vi "horizon_line.vi"(4 "center":cluster{"x":i32, "y":i32}={"x"=51, "y"=51}, 5 "color":u32(colorbox)=16711680, 6 "size":i32=40, 10 "pict in":picture) -> (3 "new out":picture)   [LabVIEW 2011]
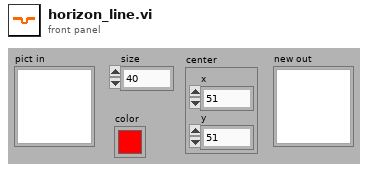
[diagram p1: front panel]
types:
  T1 = cluster{"Width":u16, "Style":enum32{"Solid", "Dash", "Dot", "DashDot", "DashDotDot"}}
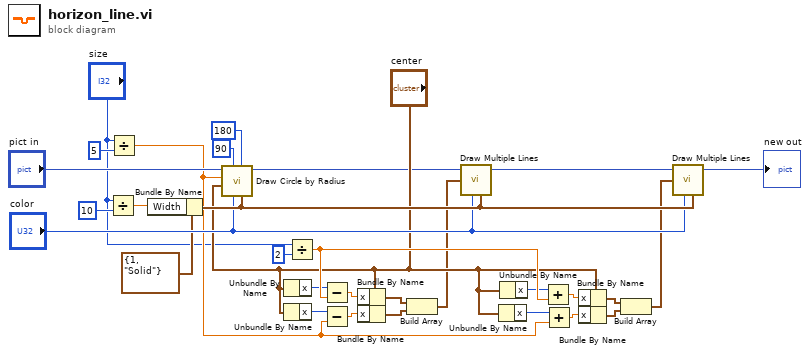
[diagram p0: block diagram]
diagram:
  n1 = Divide(x="size", y=10) -> (x/y=w8:dbl)
  n2 = Divide(x="size", y=5) -> (x/y=w2:dbl)
  n3 = Bundle By Name(cluster=T1 {"Width"=1, "Style"=enum."Solid"} ("pen"), "Width"=w8) -> (w31:T1)
  n4 = call <vilib>:"Draw Circle by Radius.vi"("pen"=w31, "arc size(360)"=i16 180, "color(black)"="color", "start angle(0)"=i16 90, "pixel center"="center", "radius"=w2, "picture"="pict in") -> ("new picture"=w10:picture)  [unwired: 4 in]
  n5 = Unbundle By Name("center") -> ("x"=w17:i32)
  n6 = Unbundle By Name("center") -> ("x"=w14:i32)
  n7 = Divide(x="size", y=2) -> (x/y=w28:dbl)
  n8 = Subtract(x=w17, y=w28) -> (x-y=w16:dbl)
  n9 = Subtract(x=w14, y=w2) -> (x-y=w15:dbl)
  n10 = Bundle By Name(cluster="center", "x"=w16) -> (w11:cluster{"x":i32, "y":i32})
  n11 = Bundle By Name(cluster="center", "x"=w15) -> (w12:cluster{"x":i32, "y":i32})
  n12 = Build Array(w11, w12) -> (w13:cluster{"x":i32, "y":i32}[])
  n13 = call <vilib>:"Draw Multiple Lines.vi"("picture"=w10, "line endpoints"=w13, "color(black)"="color", "pen"=w31) -> ("new picture"=w19:picture)  [unwired: 5 in]
  n14 = Unbundle By Name("center") -> ("x"=w23:i32)
  n15 = Unbundle By Name("center") -> ("x"=w21:i32)
  n16 = Add(x=w21, y=w28) -> (x+y=w22:dbl)
  n17 = Add(x=w23, y=w2) -> (x+y=w29:dbl)
  n18 = Bundle By Name(cluster="center", "x"=w22) -> (w25:cluster{"x":i32, "y":i32})
  n19 = Bundle By Name(cluster="center", "x"=w29) -> (w24:cluster{"x":i32, "y":i32})
  n20 = Build Array(w25, w24) -> (w26:cluster{"x":i32, "y":i32}[])
  n21 = call <vilib>:"Draw Multiple Lines.vi"("picture"=w19, "line endpoints"=w26, "color(black)"="color", "pen"=w31) -> ("new picture"=→"new out":picture)  [unwired: 5 in]
